vi "Initialise.vi"(8 "error in (no error)":errorcluster, 9 "Common":T1, 10 "Renderer":u32, 11 "Ship in":refnum<class "Ship.lvclass">) -> (0 "error out":errorcluster, 3 "Ship out":refnum<class "Ship.lvclass">)   [LabVIEW 2026, in "Ship.lvclass"]
uses:
  Ship.lvclass
  C:/dev/LabVIEW/LabMelee/Source/Application Specific/Element/Element.lvclass
  Config.ctl
  Ship.lvclass/Ship.ctl
  Re-use Libraries/Vector 2D/Vector 2D.lvclass
  Control State/Control State.lvclass
  Element/Element.lvclass
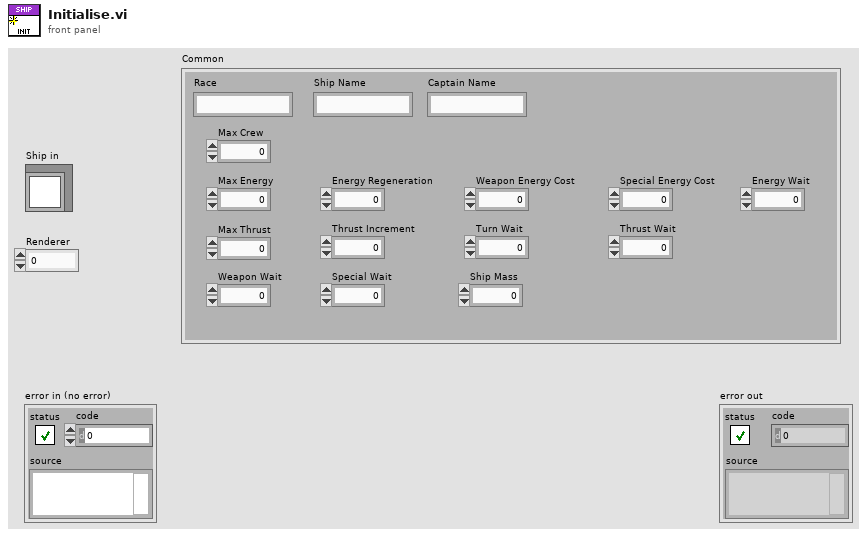
[diagram p1: front panel]
types:
  T1 = typedef "Ship.lvclass/Config.ctl" = cluster{"Race":string, "Ship Name":string, "Max Crew":i32, "Max Energy":i32, "Energy Regeneration":i32, "Weapon Energy Cost":i32, "Special Energy Cost":i32, "Energy Wait":i32, "Max Thrust":i32, "Thrust Increment":i32, "Turn Wait":i32, "Thrust Wait":i32, "Weapon Wait":i32, "Special Wait":i32, "Ship Mass":i32, "Captain Name":string}
  T2 = typedef "Constants.ctl" = cluster{"Colours":cluster{"OK":u32, "Warning":u32, "Error":u32, "Red":u32, "Green":u32, "Blue":u32, "Yellow":u32, "Health":u32, "Energy":u32}, "System":cluster{"Target Frames Second":dbl, "Windows Size":refnum<class "Vector 2D.lvclass">, "World Size":refnum<class "Vector 2D.lvclass">, "Battle Area Size":refnum<class "Vector 2D.lvclass">, "Sidebar Width":sgl, "SC2 Frame Rate [Seconds/Frame]":sgl, "Sidebar Player 2 Y Offset":sgl}, "Game":cluster{"Maximum Asteroids":i32, "Max Energy":i32, "Max Crew":i32, "Maximum Stars":i32}}
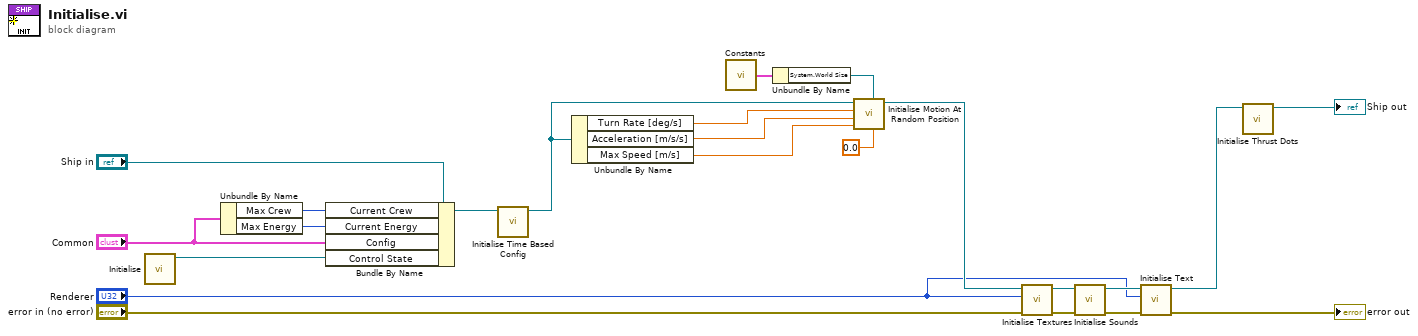
[diagram p0: block diagram]
diagram:
  n1 = call "Initialise.vi"() -> ("Control State out"=w13:refnum<class "Control State.lvclass">)  [unwired: 11 in]
  n2 = Unbundle By Name("Common") -> ("Max Crew"=w2:i32, "Max Energy"=w1:i32)
  n3 = Bundle By Name(cluster="Ship in", "Current Crew"=w2, "Current Energy"=w1, "Config"="Common", "Control State"=w13) -> (w11:refnum<class "Ship.lvclass">)
  n4 = call "Initialise Time Based Config.vi"("Ship in"=w11) -> ("Ship out"=w10:refnum<class "Ship.lvclass">)  [unwired: 10 in]
  n5 = Unbundle By Name(w10) -> ("Turn Rate [deg/s]"=w21:sgl, "Acceleration [m/s/s]"=w14:sgl, "Max Speed [m/s]"=w5:sgl)
  n6 = call "Constants.vi"() -> ("Constants"=w23:T2)
  n7 = Unbundle By Name(w23) -> ("System.World Size"=w22:refnum<class "Vector 2D.lvclass">)
  n8 = call "Initialise Motion At Random Position.vi"("Initial Velocity [m/s]"=sgl 0.0 ("Initial Heading [deg]"), "Field Size"=w22, "Maximum Velocity [m/s]"=w5, "Acceleration [m/s/s]"=w14, "Turn Rate [deg/s]"=w21, "Element in"=w10) -> ("Element out"=w9:refnum<class "Ship.lvclass">)  [unwired: 5 in]
  n9 = call "Initialise Textures.vi"("error in (no error)"="error in (no error)", "Renderer"="Renderer", "Ship in"=w9) -> ("error out"=w16:errorcluster, "Ship out"=w17:refnum<class "Ship.lvclass">)  [unwired: 7 in]
  n10 = call "Initialise Sounds.vi"("error in (no error)"=w16, "Ship in"=w17) -> ("error out"=w18:errorcluster, "Ship out"=w19:refnum<class "Ship.lvclass">)  [unwired: 8 in]
  n11 = call "Initialise Text.vi"("error in (no error)"=w18, "Renderer"="Renderer", "Ship in"=w19) -> ("error out"=→"error out":errorcluster, "Ship out"=w8:refnum<class "Ship.lvclass">)  [unwired: 7 in]
  n12 = call "Initialise Thrust Dots.vi"("Ship in"=w8) -> ("Ship out"=→"Ship out":refnum<class "Ship.lvclass">)  [unwired: 10 in]
